vi "test.vi"() -> ()   [LabVIEW 2009]
panel:
  in  "Failed Tests":i32(listbox)
  in  "VIs not loadable":i32(listbox)
  out "error type":enum16{"fatal", "non-fatal", "warning"}(ring)
  in  "VIs without test coverage":i32(listbox)
  out "error out":errorcluster
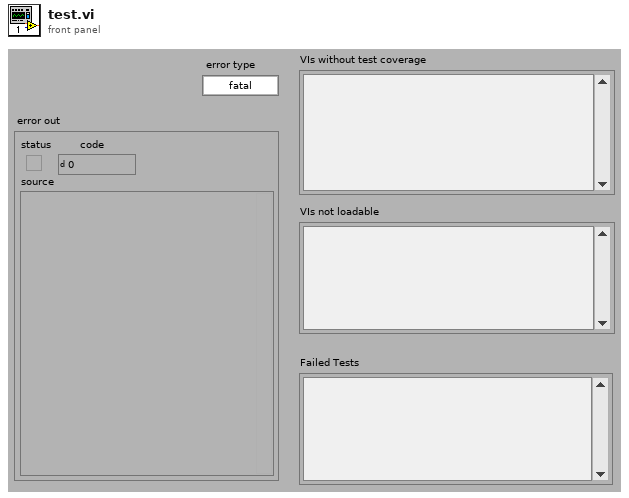
[diagram p1: front panel]
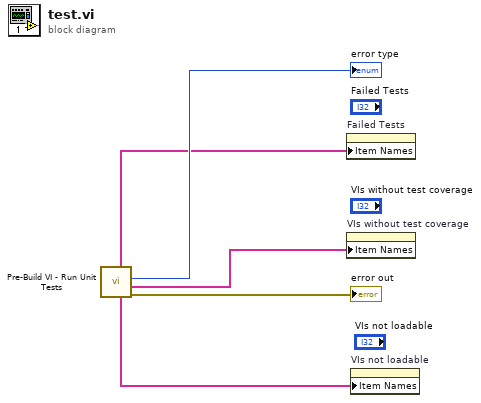
[diagram p0: block diagram]
diagram:
  n1 = call "Pre-Build VI - Run Unit Tests.vi"() -> ("error out"=→"error out":errorcluster, "VIs without test coverage"=w4:string[], "error type"=→"error type":enum16{"fatal", "non-fatal", "warning"}, "VIs not loadable"=w2:string[], "Failed Tests"=w1:string[])  [unwired: 7 in]
  n2 = property on="Failed Tests" class="ListBox (strict)"("Item Names"=w1) -> ()  [unwired: 2 in, 2 out]
  n3 = property on="VIs without test coverage" class="ListBox (strict)"("Item Names"=w4) -> ()  [unwired: 2 in, 2 out]
  n4 = property on="VIs not loadable" class="ListBox (strict)"("Item Names"=w2) -> ()  [unwired: 2 in, 2 out]
